vi "new_file.vi"() -> ()   [LabVIEW 2020]
panel:
  in  "Boolean":bool
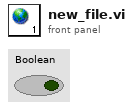
[diagram p1: front panel]
diagram:
